vi "PLC_CODMn 获取加标回收数据.vi"() -> (3 "测量数据区":T1)   [LabVIEW 2016, in "质控单元V4.lvlib"]
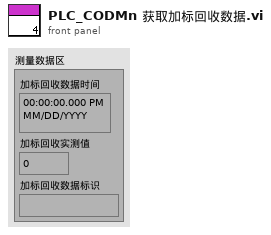
[diagram p1: front panel]
types:
  T1 = cluster{"加标回收数据时间":timestamp, "加标回收实测值":sgl, "加标回收数据标识":string}
  T2 = cluster{"因子编码":u32, "单位":u16, "标样参考值":sgl, "水样数据时间":timestamp, "水样实测值":sgl, "水样数据标识":string, "标样数据时间":timestamp, "标样实测值":sgl, "标样数据标识":string, "空白数据时间":timestamp, "空白实测值":sgl, "空白数据标识":string, "零点核查数据时间":timestamp, "零点核查实测值":sgl, "零点核查数据标识":string, "跨度核查数据时间":timestamp, "跨度核查实测值":sgl, "跨度核查数据标识":string, "加标回收数据时间":timestamp, "加标回收实测值":sgl, "加标回收数据标识":string, "平行样数据时间":timestamp, "平行样实测值":sgl, "平行样数据标识":string}
  T3 = cluster{"水样数据时间":timestamp, "水样实测值":sgl, "水样数据标识":string}
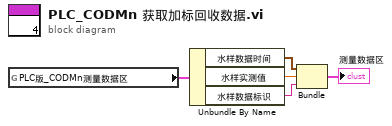
[diagram p0: block diagram]
diagram:
  n1 = global read "系统交互.vi" "PLC版_CODMn测量数据区"() -> (w5:T2)
  n2 = Unbundle By Name(w5) -> ("水样数据时间"=w4:timestamp, "水样实测值"=w3:sgl, "水样数据标识"=w2:string)
  n3 = Bundle("水样数据时间"=w4, "水样实测值"=w3, "水样数据标识"=w2) -> (→"测量数据区":T3)  [unwired: 1 in]
